vi "Actor Core.vi"(8 "error in":errorcluster, 11 "Storage in":refnum<class "Storage.lvclass">) -> (0 "error out":errorcluster, 3 "Actor out":refnum<class "Actor.lvclass">)   [LabVIEW 2015, in "AMS UI.lvlib" / "Storage.lvclass"]
doc: "(<B>Filename</B>: Actor Framework.lvlib:Actor.lvclass:Actor Core.vi)\n\nReceives messages to the actor, reacts to them, and initiates any error handling that may shut the actor down.\n\nDescendant classes may override this VI to append parallel tasks for the actor to complete while it handles messages. Overrides use the Call Parent Method node."
uses:
  Storage.lvclass
  <vilib>/ActorFramework/Actor/Actor.lvclass
  Storage.lvclass/Storage.ctl
  Storage Messages/Indicate Valves Msg/Indicate Valves Msg.lvclass/Indicate Valves Msg.ctl
  <vilib>/ActorFramework/Message Enqueuer/Message Enqueuer.lvclass/Message Enqueuer.ctl
  <vilib>/ActorFramework/Message Enqueuer/Enqueue.vi
  <vilib>/ActorFramework/Message Priority Queue/Priority Enqueue.vi
  AMS Gas Actor/AMS Gas Actor.lvclass
  Storage Messages/Indicate Valves Msg/Indicate Valves Msg.lvclass
  Storage Messages/Indicate Tubes Msg/Indicate Tubes Msg.lvclass
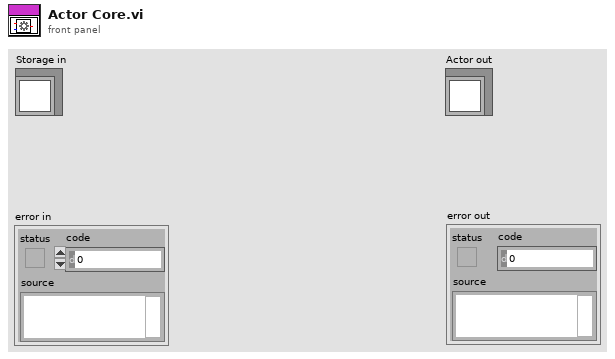
[diagram p1: front panel]
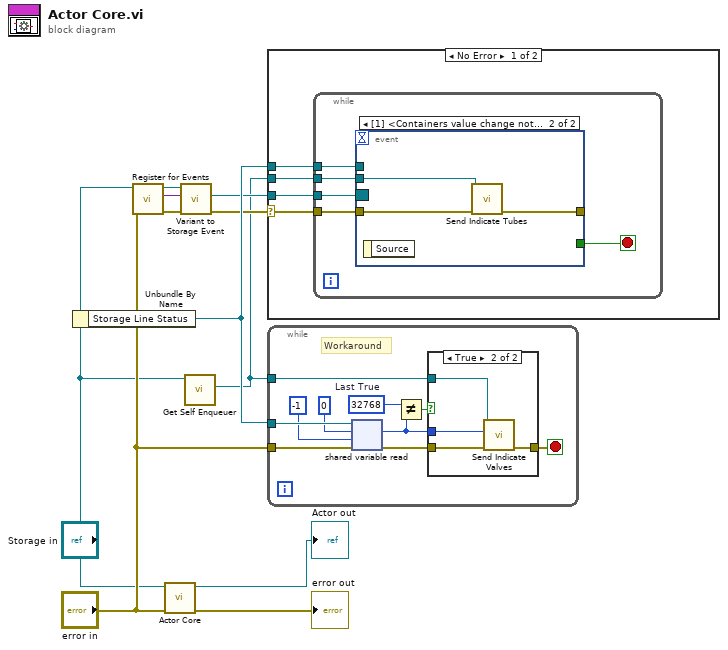
[diagram p0: block diagram]
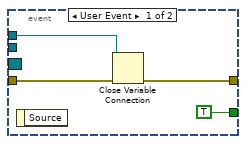
[diagram p3: hidden frame]
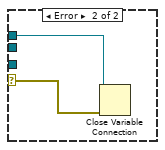
[diagram p4: hidden frame]
diagram:
  n1 = Unbundle By Name("Storage in") -> ("Storage Line Status"=w9:refnum<k21>)
  n2 = call-dynamic "Register for Events.vi"("error in (no error)"="error in", "Storage in"="Storage in") -> ("error out"=w3:errorcluster, "Event Registration Refnum"=w8:variant, "Storage out"=w4:refnum<class "Storage.lvclass">)  [unwired: 7 in]
  n3 = call-parent "Actor Core.vi"("error in"="error in", "Actor in"="Storage in") -> ("error out"=→"error out":errorcluster, "Actor out"=→"Actor out":refnum<class "Actor.lvclass">)  [unwired: 8 in]
  n4 = call "Variant to Storage Event.vi"("error in (no error)"=w3, "variant"=w8, "Storage in"=w4) -> ("error out"=w2:errorcluster, "Event Registration Refnum"=w5:refnum<event-registration>)  [unwired: 6 in, 1 out]
  n5 = call-dynamic "Get Self Enqueuer.vi"("eActor in"="Storage in") -> ("Actor Framework:Message Enqueuer"=w1:refnum<class "Message Enqueuer.lvclass">)  [unwired: 9 in, 1 out]
  n6 = case shown="No Error" w2 {
    selector: w2 -> [w13 w28]
    tunnel: w5 -> [w15 _]
    tunnel: w9 -> [w14 w29]
    tunnel: w1 -> [w12 _]
    frame No Error {
      n7 = while {
        tunnel: w15 -> [w20]
        tunnel: w14 -> [w19]
        tunnel: w13 -> [w18]
        tunnel: w12 -> [w16]
        stop <- w17 stop-if-true
        n8 = event shown="[1] <Containers value change notification>: User Event" {
          selector: w20 -> [_ _]
          dyn-events: _ -> [_ _]
          timeout: _ -> [_ _]
          tunnel: w19 -> [w23 _]
          tunnel: w18 -> [w24 w27]
          tunnel: [w22 w25] -> _
          tunnel: [TRUE _] -> w17
          tunnel: w16 -> [_ w26]
          event User Event {
            n9 = event-data() -> ()  [unwired: 1 in, 1 out]
            n10 = Close Variable Connection(8:w24, 11:w23) -> (0:w22:errorcluster)
          }
          event User Event {
            n11 = event-data() -> ()  [unwired: 1 in, 1 out]
            n12 = call "Send Indicate Tubes.vi"("error in (no error)"=w27, "Message Enqueuer"=w26) -> ("error out"=w25:errorcluster)  [unwired: 8 in, 1 out]
          }
        }
      }
    }
    frame Error {
      n13 = Close Variable Connection(8:w28, 11:w29) -> ()  [unwired: 1 out]
    }
  }
  n14 = while {
    tunnel: "error in" -> [w38]
    tunnel: w9 -> [w37]
    tunnel: w1 -> [w30]
    stop <- w39 stop-if-true
    w31 = u16 32768  # Last True
    # "Workaround"
    n15 = shared-variable-read(w37, w38, u16 0, -1 ("timeout ms")) -> (w35:errorcluster, w32:u16)  [unwired: 3 out]
    n16 = Not Equal?(x=w31, y=w32) -> (x != y?=w33:bool)
    n17 = case shown="True" w33 {
      tunnel: [w40 w44] -> w39
      tunnel: w32 -> [_ w43]
      tunnel: w35 -> [w40 w42]
      tunnel: w30 -> [_ w41]
      frame False {
        # "The value is\nfor refreshing\npurposes.\nIgnore"
      }
      frame True {
        n18 = call "Send Indicate Valves.vi"("error in (no error)"=w42, "Numeric"=w43, "Message Enqueuer"=w41) -> ("error out"=w44:errorcluster)  [unwired: 7 in, 1 out]
      }
    }
  }
